vi "Build HTML Destination.vi"(8 "Error In":errorcluster, 10 "Hierarchy Folders":string[](array[string]), 11 "Root Destination":path=path "") -> (0 "Error Out":errorcluster, 3 "HTML Destination":path)   [LabVIEW 2018, in "Scripts.lvlib"]
uses:
  Scripts.lvlib
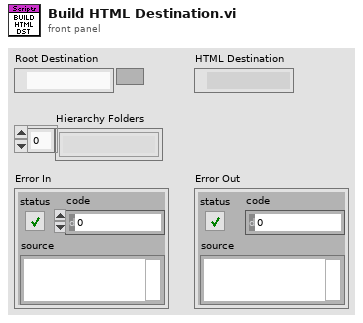
[diagram p1: front panel]
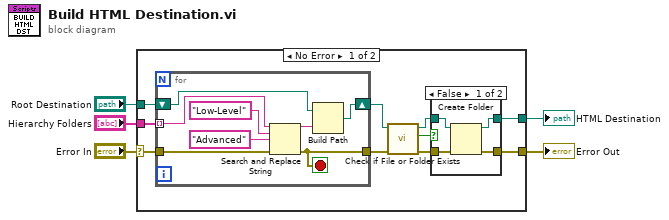
[diagram p0: block diagram]
diagram:
  n1 = case shown="No Error" "Error In" {
    selector: "Error In" -> [w6 w30]
    tunnel: "Hierarchy Folders" -> [w15 _]
    tunnel: "Root Destination" -> [w14 _]
    tunnel: [w8 w30] -> w3
    tunnel: [w7 _] -> w2
    frame No Error {
      n2 = for {
        tunnel: w15 -> [w27] mode=indexing
        shift-right: [w28] -> w10
        shift-left: w14 -> [w29]
        tunnel: w6 -> [w24]
        tunnel: [w23] -> w9
        stop <- w23 stop-if-true
        n3 = Search and Replace String(input string=w27, search string="Low-Level" ("substring (\"\")"), replace string="Advanced" ("replace string (\"\")"), error in=w24) -> (result string=w22:string, error out=w23:errorcluster)  [unwired: 4 in, 2 out]
        n4 = Build Path(base path=w29, name or relative path=w22) -> (appended path=w28:path)
      }
      n5 = call <vilib>:"Check if File or Folder Exists.vi"("error in (no error)"=w9, "path"=w10) -> ("error out"=w13:errorcluster, "file or folder exists?"=w11:bool, "dup path"=w12:path)  [unwired: 7 in]
      n6 = case shown="False" w11 {
        tunnel: w12 -> [w19 w21]
        tunnel: [w18 w21] -> w7
        tunnel: w13 -> [w16 w20]
        tunnel: [w17 w20] -> w8
        frame False {
          n7 = Create Folder(path (use dialog)=w19, error in=w16) -> (created path=w18:path, error out=w17:errorcluster)  [unwired: 1 in, 1 out]
        }
        frame True {
        }
      }
    }
    frame Error {
    }
  }
  "HTML Destination" <- w2
  "Error Out" <- w3
